vi "GetControlReferenceByName.vi"(10 "Telemetry Data":string, 11 "Cluster in":refnum<vi>) -> (2 "Boolean":bool, 3 "Control out":refnum<vi>)   [LabVIEW 2016]
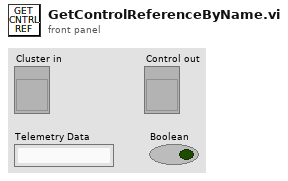
[diagram p1: front panel]
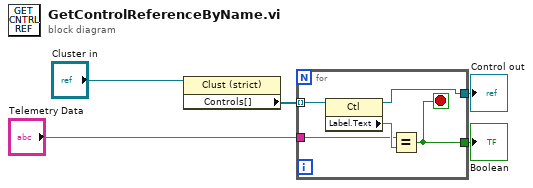
[diagram p0: block diagram]
diagram:
  n1 = property on="Property Node" class="Clust (strict)"(reference="Cluster in") -> ("Controls[]"=w1:refnum<vi>[])  [unwired: 1 in, 2 out]
  n2 = for {
    tunnel: w1 -> [w10] mode=indexing
    tunnel: [w9] -> w5
    tunnel: "Telemetry Data" -> [w7]
    tunnel: [w6] -> w4
    stop <- w6 stop-if-true
    n3 = property on="Property Node" class="Ctl"(reference=w10) -> (reference out=w9:refnum<vi>, "Label.Text"=w8:string)  [unwired: 1 in, 1 out]
    n4 = Equal?(x=w7, y=w8) -> (x = y?=w6:bool)
  }
  "Control out" <- w5
  "Boolean" <- w4
